vi "DSF.Engine.Plugin.Create.vi"(8 "error in (no error)":errorcluster, 9 "Timing":refnum<class "DSF.Engine.Timing.lvclass">, 10 "Transceiver type":refnum<class "DSF.Engine.Transceiver.lvclass">, 11 "Transfer Groups":refnum<class "DSF.Engine.Transfer Group.lvclass">[](array[class])) -> (0 "error out":errorcluster, 3 "Plugin out":refnum<class "DSF.Engine.Plugin.lvclass">)   [LabVIEW 2017, in "DSF.Engine.lvlib" / "DSF.Engine.Plugin.lvclass"]
uses:
  DSF.Engine.Plugin.lvclass
  Timing/DSF.Engine.Timing.lvclass
  Transceiver/DSF.Engine.Transceiver.lvclass
  Transfer/DSF.Engine.Transfer Group.lvclass
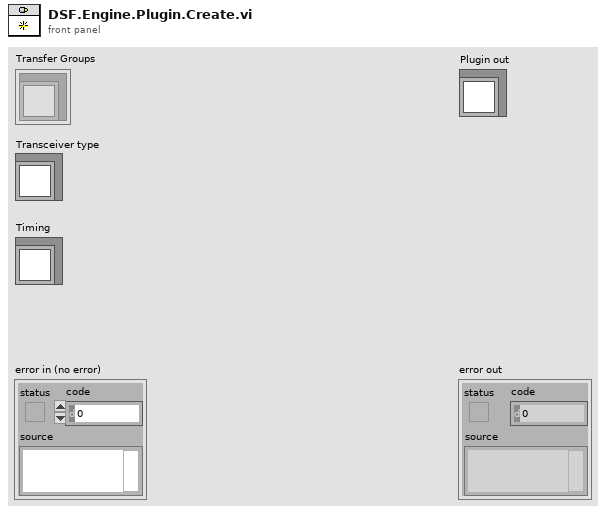
[diagram p1: front panel]
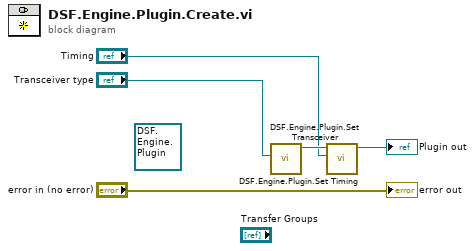
[diagram p0: block diagram]
diagram:
  (unwired) refnum<class "DSF.Engine.Plugin.lvclass"> refnum ("Plugin in")
  n1 = call "DSF.Engine.Plugin.Set Transceiver.vi"("Transceiver"="Transceiver type") -> ("Plugin out"=w4:refnum<class "DSF.Engine.Plugin.lvclass">)  [unwired: 10 in]
  n2 = call "DSF.Engine.Plugin.Set Timing.vi"("Timing"="Timing", "Plugin in"=w4) -> ("Plugin out"=→"Plugin out":refnum<class "DSF.Engine.Plugin.lvclass">)  [unwired: 9 in]
  "error out" <- "error in (no error)"
